vi "create list of files.vi"(0 "Path (folder) 2":path caption="Path (multiple)", 2 "Single file (T)":bool=TRUE, 5 "Path (file)":path caption="Path (single)", 7 "Match pattern:":string, 9 "File extension:":string, 12 "Subfolders?":bool=TRUE, 13 "Overwrite .csv files:":bool=TRUE) -> (4 "Array of files to be converted":path[](array[path]), 6 "Array of .csv":path[](array[path]), 8 "Array of .metadat.csv":path[](array[path]), 14 "Path for read me":path, 15 "Files to convert to CSV:":string)   [LabVIEW 2010]
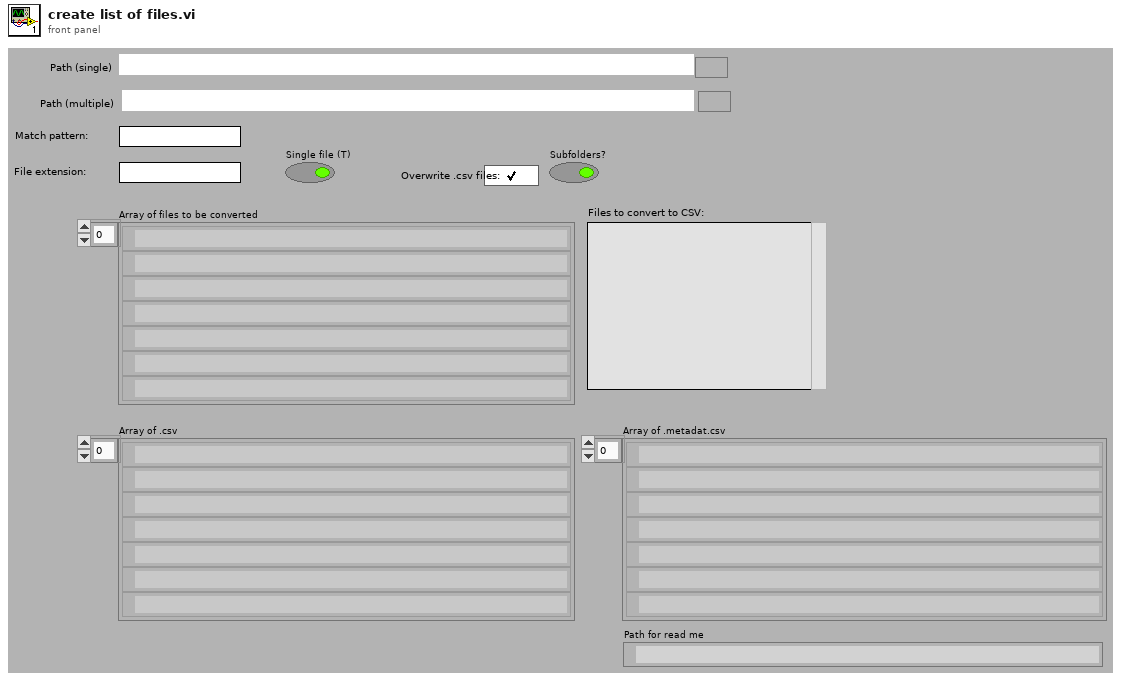
[diagram p1: front panel]
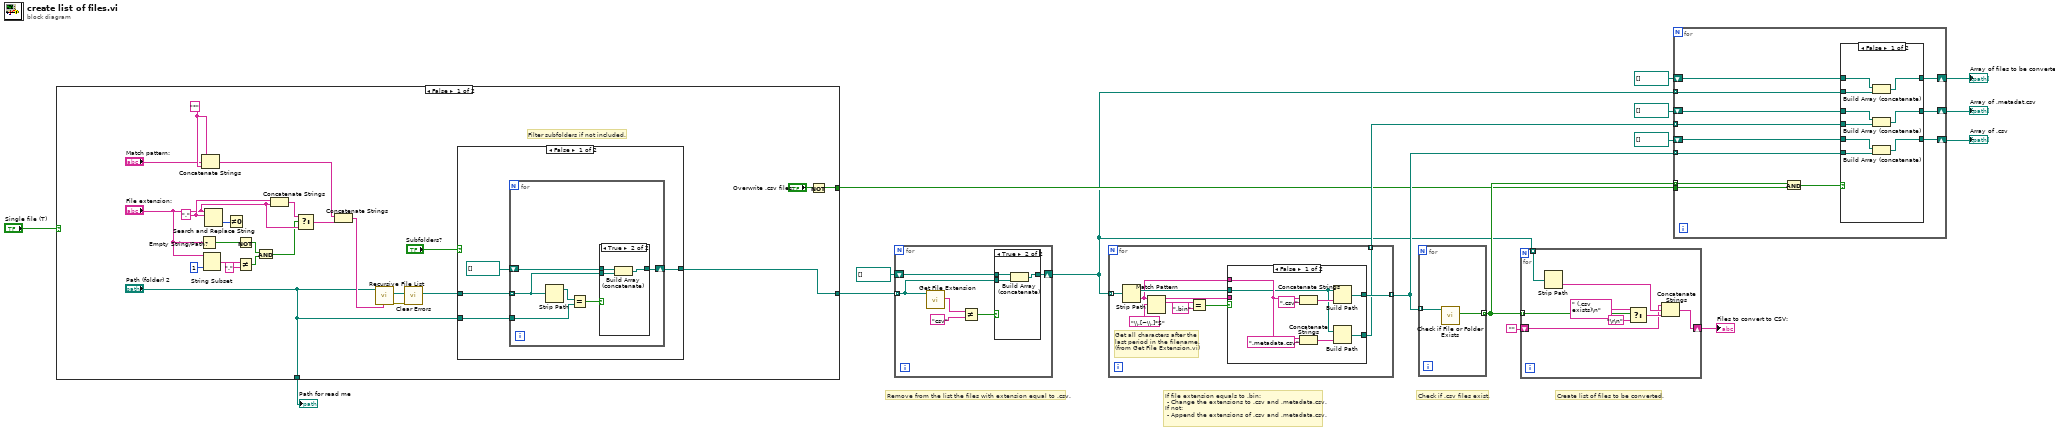
[diagram p0: block diagram]
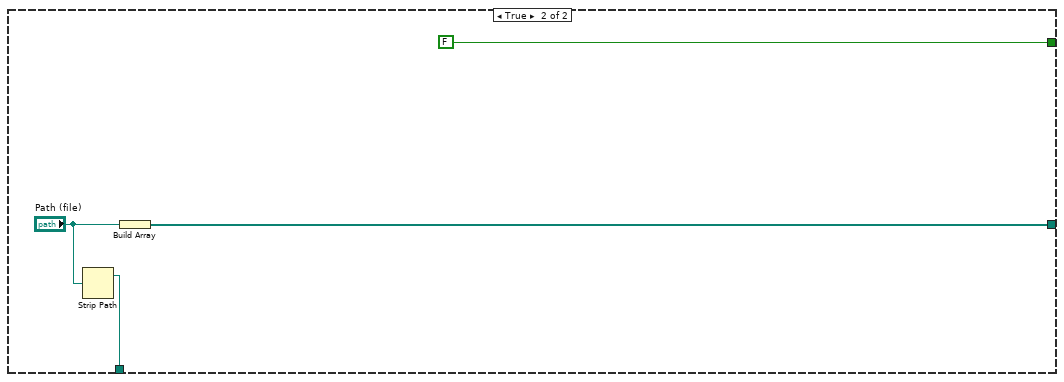
[diagram p6: hidden frame]
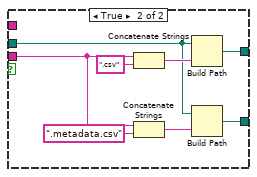
[diagram p7: hidden frame]
diagram:
  # "Remove from the list the files with extension equal to .csv."
  # "Create list of files to be converted."
  # "Check if .csv files exist."
  # "If file extension equals to .bin:\n - Change the extensions to .csv and .metadata.csv.\nIf not:\n - Append the extensions of .csv and .metadata.csv."
  n1 = case shown="False" "Single file (T)" {
    tunnel: [w28 w59] -> w3
    tunnel: ["Path (folder) 2" w57] -> w14
    tunnel: [w31 FALSE ("Skip if file exist:")] -> w4
    frame False {
      w37 = "*" ("string")
      w34 = "." ("search string")
      # "Filter subfolders if not included."
      n2 = Empty String/Path?(string/path="File extension:") -> (empty?=w25:bool)
      n3 = Concatenate Strings(w37, "Match pattern:", w37) -> (w39:string)
      n4 = String Subset(string="File extension:", length (rest)=1 ("length (rest)")) -> (substring=w22:string)  [unwired: 1 in]
      n5 = Search and Replace String(input string="File extension:", search string=w34) -> (offset past replacement=w33:i32)  [unwired: 6 in, 3 out]
      n6 = Not Equal To 0?(x=w33) -> ()  [unwired: 1 out]
      n7 = Not(x=w25) -> (.not. x?=w19:bool)
      n8 = Not Equal?(x=w22, y=".") -> (x != y?=w20:bool)
      n9 = And(x=w19, y=w20) -> (x .and. y?=w18:bool)
      n10 = Concatenate Strings(w34, "File extension:") -> (w35:string)
      n11 = Select(t=w35, s=w18, f="File extension:") -> (s? t:f=w38:string)
      n12 = Concatenate Strings(w39, w38) -> (w40:string)
      n13 = call <vilib>:"Recursive File List.vi"("pattern"=w40, "Folder Path"="Path (folder) 2") -> ("error out"=w26:errorcluster, "All Files in Dir"=w30:path[])  [unwired: 5 in, 3 out]
      n14 = call <vilib>:"Clear Errors.vi"("error in (no error)"=w26) -> ()  [unwired: 6 in, 1 out]
      n15 = case shown="False" "Subfolders?" {
        tunnel: w30 -> [w44 w55]
        tunnel: "Path (folder) 2" -> [w43 _]
        tunnel: [w41 w55] -> w28
        frame False {
          n16 = for {
            tunnel: w44 -> [w45] mode=indexing
            tunnel: w43 -> [w49]
            shift-right: [w47] -> w41
            shift-left: path[] [] -> [w46]
            n17 = Strip Path(path=w45) -> (stripped path=w50:path)  [unwired: 1 out]
            n18 = Equal?(x=w50, y=w49) -> (x = y?=w48:bool)
            n19 = case shown="True" w48 {
              tunnel: [w51 w53] -> w47
              tunnel: w46 -> [w51 w54]
              tunnel: w45 -> [_ w52]
              frame False {
              }
              frame True {
                n20 = Build Array (concatenate)(w54, w52) -> (w53:path[])
              }
            }
          }
        }
        frame True {
        }
      }
      n21 = Not(x="Overwrite .csv files:") -> (.not. x?=w31:bool)
    }
    frame True {
      n22 = Strip Path(path="Path (file)") -> (stripped path=w57:path)  [unwired: 1 out]
      n23 = Build Array("Path (file)") -> (w59:path[])
    }
  }
  "Path for read me" <- w14
  n24 = for {
    tunnel: w3 -> [w62] mode=indexing
    shift-right: [w64] -> w1
    shift-left: path[] [] ("All Files in Dir") -> [w63]
    n25 = call <vilib>:"Get File Extension.vi"("file"=w62) -> ("lowercase file extension"=w61:string)  [unwired: 7 in, 3 out]
    n26 = Not Equal?(x=w61, y="csv" ("regular expression")) -> (x != y?=w65:bool)
    n27 = case shown="True" w65 {
      tunnel: [w66 w69] -> w64
      tunnel: w62 -> [_ w68]
      tunnel: w63 -> [w66 w67]
      frame False {
      }
      frame True {
        n28 = Build Array (concatenate)(w67, w68) -> (w69:path[])
      }
    }
  }
  n29 = for {
    tunnel: w1 -> [w78] mode=indexing
    tunnel: [w77] -> w12 mode=indexing
    tunnel: [w74] -> w13 mode=indexing
    # "Get all characters after the\nlast period in the filename.\n(from Get File Extension.vi)"
    n30 = Strip Path(path=w78) -> (stripped path=w75:path, name=w71:string)
    n31 = Match Pattern(string=w71, regular expression="\\.[~\\.]*$") -> (before substring=w76:string, match substring=w73:string)  [unwired: 3 out]
    n32 = Equal?(x=w73, y=".bin") -> (x = y?=w70:bool)
    n33 = case shown="False" w70 {
      tunnel: [w81 w93] -> w77
      tunnel: w76 -> [_ w91]
      tunnel: w75 -> [w82 w89]
      tunnel: [w80 w88] -> w74
      tunnel: w71 -> [w83 _]
      frame False {
        n34 = Concatenate Strings(w83, ".csv" ("string")) -> (w86:string)
        n35 = Concatenate Strings(w83, ".metadata.csv" ("string")) -> (w84:string)
        n36 = Build Path(base path=w82, name or relative path=w86) -> (appended path=w81:path)
        n37 = Build Path(base path=w82, name or relative path=w84) -> (appended path=w80:path)
      }
      frame True {
        n38 = Concatenate Strings(w91, ".csv" ("string")) -> (w94:string)
        n39 = Concatenate Strings(w91, ".metadata.csv" ("string")) -> (w90:string)
        n40 = Build Path(base path=w89, name or relative path=w94) -> (appended path=w93:path)
        n41 = Build Path(base path=w89, name or relative path=w90) -> (appended path=w88:path)
      }
    }
  }
  n42 = for {
    tunnel: w12 -> [w97] mode=indexing
    tunnel: [w96] -> w11 mode=indexing
    n43 = call <vilib>:"Check if File or Folder Exists.vi"("path"=w97) -> ("file or folder exists?"=w96:bool)  [unwired: 8 in, 2 out]
  }
  n44 = for {
    tunnel: w1 -> [w105] mode=indexing
    tunnel: w11 -> [w104] mode=indexing
    shift-right: [w99] -> w17
    shift-left: "" -> [w98]
    n45 = Strip Path(path=w105) -> (name=w100:string)  [unwired: 1 out]
    n46 = Select(t=" (.csv exists)\n" ("name"), s=w104, f="\r\n") -> (s? t:f=w103:string)
    n47 = Concatenate Strings(w98, w100, w103) -> (w99:string)
  }
  "Files to convert to CSV:" <- w17
  n48 = for {
    tunnel: w1 -> [w115] mode=indexing
    tunnel: w13 -> [w113] mode=indexing
    tunnel: w12 -> [w112] mode=indexing
    tunnel: w11 -> [w117] mode=indexing
    shift-right: [w114] -> w7
    shift-left: path[] [] -> [w116]
    shift-right: [w108] -> w6
    shift-left: path[] [] -> [w111]
    shift-right: [w109] -> w5
    shift-left: path[] [] -> [w110]
    tunnel: w4 -> [w106]
    n49 = And(x=w117, y=w106) -> (x .and. y?=w107:bool)
    n50 = case shown="False" w107 {
      tunnel: w115 -> [w125 _]
      tunnel: w116 -> [w126 w129]
      tunnel: [w124 w129] -> w114
      tunnel: w113 -> [w122 _]
      tunnel: w111 -> [w121 w128]
      tunnel: [w123 w128] -> w108
      tunnel: w112 -> [w119 _]
      tunnel: w110 -> [w120 w127]
      tunnel: [w118 w127] -> w109
      frame False {
        n51 = Build Array (concatenate)(w126, w125) -> (w124:path[])
        n52 = Build Array (concatenate)(w121, w122) -> (w123:path[])
        n53 = Build Array (concatenate)(w120, w119) -> (w118:path[])
      }
      frame True {
      }
    }
  }
  "Array of .csv" <- w5
  "Array of files to be converted" <- w7
  "Array of .metadat.csv" <- w6
